vi "Main_Potential-Field_Sim.vi"() -> ()   [LabVIEW 2019]
uses:
  Ctrl/cmd_common.ctl
panel:
  in  "tap":enum32{"Main", "Data"}(tab)
  in  "set goal point":bool
  in  "set start point":bool
  in  "calc potential map":bool
  out "Potential graph":dbl[][](graph)
  in  "Run":bool
  in  "clear":bool
  out "N of obstacles":i32(slide)=8 scale=0.0..20.0
  in  "add obstacle":bool
  in  "Finish":bool
  out "Waypoint":cluster{"rxy":cluster{"x":dbl, "y":dbl}[]}[](graph)=[{"rxy"=[{"x"=9.0, "y"=13.0}]}, {"rxy"=[{"x"=111.0, "y"=90.0}]}, {"rxy"=[{"x"=15.0, "y"=25.0}, {"x"=5.0, "y"=15.0}, {"x"=20.0, "y"=26.0}, {"x"=25.0, "y"=25.0}, {"x"=39.0, "y"=43.0}, {"x"=57.0, "y"=62.0}, {"x"=53.0, "y"=40.0}, {"x"=65.0, "y"=65.0}]}, {"rxy"=[{"x"=65.0, "y"=65.0}]}, {"rxy"=[{"x"=9.0, "y"=13.0}, {"x"=9.5, "y"=13.5}, {"x"=10.0, "y"=14.0}, {"x"=10.5, "y"=14.5}, {"x"=11.0, "y"=15.0}, {"x"=11.5, "y"=15.5}, {"x"=12.0, "y"=16.0}, {"x"=12.5, "y"=16.5}, {"x"=13.0, "y"=17.0}, {"x"=13.5, "y"=17.5}, {"x"=14.0, "y"=18.0}, {"x"=14.5, "y"=18.5}, {"x"=15.0, "y"=19.0}, {"x"=15.5, "y"=19.5}, {"x"=16.0, "y"=20.0}, {"x"=16.5, "y"=20.5}, {"x"=17.0, "y"=21.0}, {"x"=17.5, "y"=21.5}, {"x"=18.0, "y"=22.0}, {"x"=18.5, "y"=22.5}, {"x"=19.0, "y"=23.0}, {"x"=19.5, "y"=23.0}, {"x"=20.0, "y"=23.0}, {"x"=20.5, "y"=23.0}, {"x"=21.0, "y"=23.0}, {"x"=21.5, "y"=23.5}, {"x"=22.0, "y"=24.0}, {"x"=22.5, "y"=24.5}, {"x"=22.5, "y"=25.0}, {"x"=22.5, "y"=25.5}, {"x"=22.5, "y"=26.0}, {"x"=23.0, "y"=26.5}, {"x"=23.5, "y"=27.0}, {"x"=24.0, "y"=27.5}, {"x"=24.5, "y"=28.0}, {"x"=25.0, "y"=28.5}, {"x"=25.5, "y"=29.0}, {"x"=26.0, "y"=29.5}, {"x"=26.5, "y"=30.0}, {"x"=27.0, "y"=30.5}, {"x"=27.5, "y"=31.0}, {"x"=28.0, "y"=31.5}, {"x"=28.5, "y"=32.0}, {"x"=29.0, "y"=32.5}, {"x"=29.5, "y"=33.0}, {"x"=30.0, "y"=33.5}, {"x"=30.5, "y"=34.0}, {"x"=31.0, "y"=34.5}, {"x"=31.5, "y"=35.0}, {"x"=32.0, "y"=35.5}, {"x"=32.5, "y"=36.0}, {"x"=33.0, "y"=36.5}, {"x"=33.5, "y"=37.0}, {"x"=34.0, "y"=37.5}, {"x"=34.5, "y"=38.0}, {"x"=35.0, "y"=38.5}, {"x"=35.5, "y"=39.0}, {"x"=36.0, "y"=39.5}, {"x"=36.5, "y"=40.0}, {"x"=37.0, "y"=40.5}, {"x"=37.5, "y"=40.5}, {"x"=38.0, "y"=40.0}, {"x"=38.5, "y"=40.0}, {"x"=39.0, "y"=40.0}, {"x"=39.5, "y"=40.0}, {"x"=40.0, "y"=40.0}, {"x"=40.5, "y"=40.5}, {"x"=41.0, "y"=41.0}, {"x"=41.5, "y"=41.5}, {"x"=42.0, "y"=42.0}, {"x"=42.5, "y"=42.5}, {"x"=43.0, "y"=43.0}, {"x"=43.5, "y"=43.5}, {"x"=44.0, "y"=44.0}, {"x"=44.5, "y"=44.5}, {"x"=45.0, "y"=45.0}, {"x"=45.5, "y"=45.5}, {"x"=46.0, "y"=46.0}, {"x"=46.5, "y"=46.5}, {"x"=47.0, "y"=47.0}, {"x"=47.5, "y"=47.5}, {"x"=48.0, "y"=48.0}, {"x"=48.5, "y"=48.5}, {"x"=49.0, "y"=49.0}, {"x"=49.5, "y"=49.5}, {"x"=50.0, "y"=50.0}, {"x"=50.5, "y"=50.5}, {"x"=51.0, "y"=51.0}, {"x"=51.5, "y"=51.5}, {"x"=52.0, "y"=52.0}, {"x"=52.5, "y"=52.5}, {"x"=53.0, "y"=53.0}, {"x"=53.5, "y"=53.5}, {"x"=54.0, "y"=54.0}, {"x"=54.5, "y"=54.5}, {"x"=55.0, "y"=55.0}, {"x"=55.5, "y"=55.5}, {"x"=56.0, "y"=56.0}, {"x"=56.5, "y"=56.5}, {"x"=57.0, "y"=57.0}, {"x"=57.5, "y"=57.5}, {"x"=58.0, "y"=58.0}, {"x"=58.5, "y"=58.5}, {"x"=59.0, "y"=59.0}, {"x"=59.5, "y"=59.5}, {"x"=60.0, "y"=60.0}, {"x"=60.5, "y"=60.5}, {"x"=61.0, "y"=61.0}, {"x"=61.5, "y"=61.5}, {"x"=62.0, "y"=62.0}, {"x"=62.5, "y"=62.5}, {"x"=63.0, "y"=63.0}, {"x"=63.5, "y"=62.5}, {"x"=64.0, "y"=62.0}, {"x"=64.5, "y"=62.0}, {"x"=65.0, "y"=62.0}, {"x"=65.5, "y"=62.0}, {"x"=66.0, "y"=62.0}, {"x"=66.5, "y"=62.5}, {"x"=67.0, "y"=63.0}, {"x"=67.5, "y"=63.5}, {"x"=68.0, "y"=64.0}, {"x"=68.5, "y"=64.5}, {"x"=69.0, "y"=65.0}, {"x"=69.5, "y"=65.5}, {"x"=70.0, "y"=66.0}, {"x"=70.5, "y"=66.5}, {"x"=71.0, "y"=67.0}, {"x"=71.5, "y"=67.5}, {"x"=72.0, "y"=68.0}, {"x"=72.5, "y"=68.5}, {"x"=73.0, "y"=69.0}, {"x"=73.5, "y"=69.5}, {"x"=74.0, "y"=70.0}, {"x"=74.5, "y"=70.5}, {"x"=75.0, "y"=71.0}, {"x"=75.5, "y"=71.5}, {"x"=76.0, "y"=72.0}, {"x"=76.5, "y"=72.5}, {"x"=77.0, "y"=73.0}, {"x"=77.5, "y"=73.5}, {"x"=78.0, "y"=74.0}, {"x"=78.5, "y"=74.5}, {"x"=79.0, "y"=75.0}, {"x"=79.5, "y"=75.5}, {"x"=80.0, "y"=76.0}, {"x"=80.5, "y"=76.5}, {"x"=81.0, "y"=77.0}, {"x"=81.5, "y"=77.5}, {"x"=82.0, "y"=78.0}, {"x"=82.5, "y"=78.5}, {"x"=83.0, "y"=79.0}, {"x"=83.5, "y"=79.5}, {"x"=84.0, "y"=80.0}, {"x"=84.5, "y"=80.5}, {"x"=85.0, "y"=81.0}, {"x"=85.5, "y"=81.5}, {"x"=86.0, "y"=82.0}, {"x"=86.5, "y"=82.5}, {"x"=87.0, "y"=83.0}, {"x"=87.5, "y"=83.5}, {"x"=88.0, "y"=84.0}, {"x"=88.5, "y"=84.5}, {"x"=89.0, "y"=85.0}, {"x"=89.5, "y"=85.5}, {"x"=90.0, "y"=86.0}, {"x"=90.5, "y"=86.5}, {"x"=91.0, "y"=87.0}, {"x"=91.5, "y"=87.5}, {"x"=92.0, "y"=88.0}, {"x"=92.5, "y"=88.5}, {"x"=93.0, "y"=89.0}, {"x"=93.5, "y"=89.5}, {"x"=94.0, "y"=90.0}, {"x"=94.5, "y"=90.0}, {"x"=95.0, "y"=90.0}, {"x"=95.5, "y"=90.0}, {"x"=96.0, "y"=90.0}, {"x"=96.5, "y"=90.0}, {"x"=97.0, "y"=90.0}, {"x"=97.5, "y"=90.0}, {"x"=98.0, "y"=90.0}, {"x"=98.5, "y"=90.0}, {"x"=99.0, "y"=90.0}, {"x"=99.5, "y"=90.0}, {"x"=100.0, "y"=90.0}, {"x"=100.5, "y"=90.0}, {"x"=101.0, "y"=90.0}, {"x"=101.5, "y"=90.0}, {"x"=102.0, "y"=90.0}, {"x"=102.5, "y"=90.0}, {"x"=103.0, "y"=90.0}, {"x"=103.5, "y"=90.0}, {"x"=104.0, "y"=90.0}, {"x"=104.5, "y"=90.0}, {"x"=105.0, "y"=90.0}, {"x"=105.5, "y"=90.0}, {"x"=106.0, "y"=90.0}, {"x"=106.5, "y"=90.0}, {"x"=107.0, "y"=90.0}, {"x"=107.5, "y"=90.0}, {"x"=108.0, "y"=90.0}, {"x"=108.5, "y"=90.0}, {"x"=109.0, "y"=90.0}, {"x"=109.5, "y"=90.0}, {"x"=110.0, "y"=90.0}, {"x"=110.5, "y"=90.0}, {"x"=111.0, "y"=90.0}]}]
  in  "global-val":T1={"KP"=5.0, "ETA"=100.0, "AREA_WIDTH"=30.0, "Osc_Det_Len"=3}
  in  "set-val":T2={"start pt"={"x"=0, "y"=10}, "goal pt"={"x"=90, "y"=90}, "grid size"=0.5, "robot radius"=5.0, "obstacles"=[{"x"=15, "y"=25}, {"x"=5, "y"=15}, {"x"=20, "y"=26}, {"x"=25, "y"=25}]}
  out "add point":cluster{i32, i32}={65, 65}
  # "Made by Ybbaek"
  # "Potential Field Simulation"
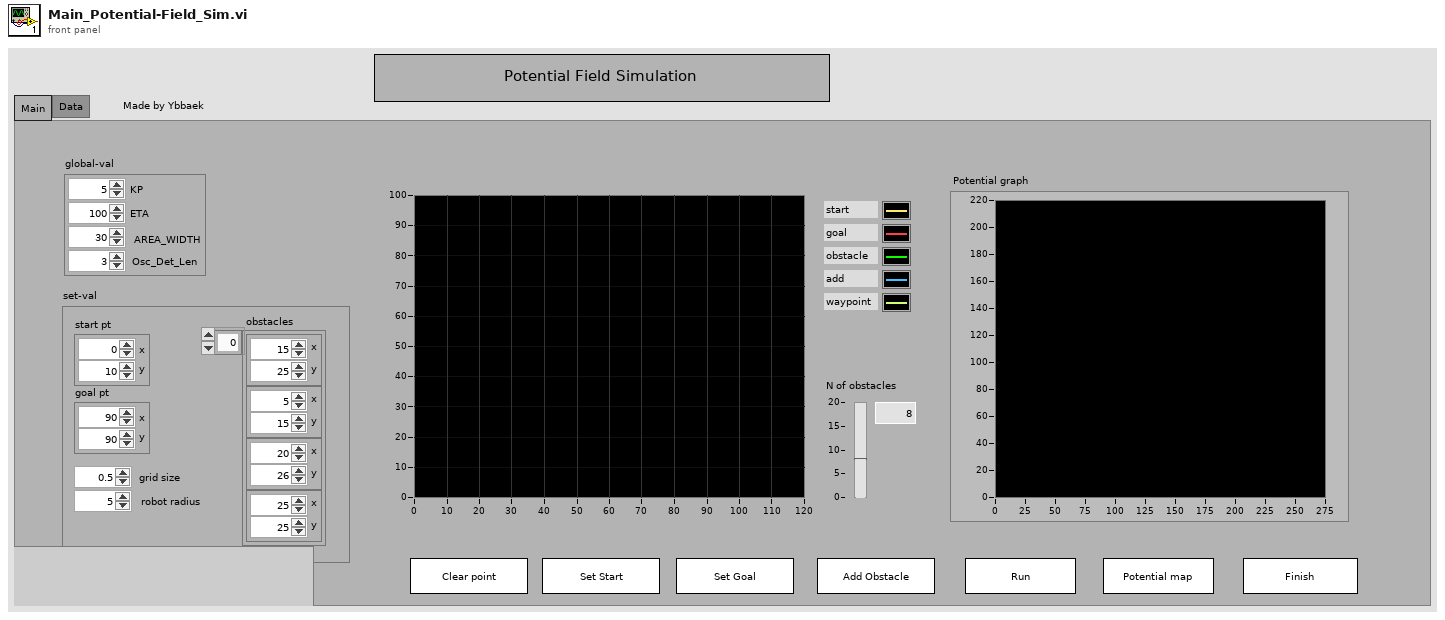
[diagram p1: front panel]
types:
  T1 = cluster{"KP":dbl, "ETA":dbl, "AREA_WIDTH":dbl, "Osc_Det_Len":u32}
  T2 = cluster{"start pt":cluster{"x":i32, "y":i32}, "goal pt":cluster{"x":i32, "y":i32}, "grid size":dbl, "robot radius":dbl, "obstacles":cluster{"x":i32, "y":i32}[]}
  T3 = typedef "cmd_common.ctl" = enum16{"read", "write"}
  T4 = cluster{"start pt":cluster{"x":i32, "y":dbl}, "goal pt":cluster{"x":i32, "y":i32}, "grid size":dbl, "robot radius":dbl, "obstacles":cluster{"x":i32, "y":i32}[]}
  T5 = typedef "NI_Matrix.lvlib/RealMatrix.ctl" = dbl[][]
  T6 = cluster{"delay":dbl, "d":dbl, "rxy":cluster{"x":dbl, "y":dbl}[], "pmap":T5}
  T7 = typedef "LVPoint32TypeDef.ctl" = cluster{"Horizontal":i32, "Vertical":i32}
  T8 = typedef "LVRectTypeDef.ctl" = cluster{"Left":i16, "Top":i16, "Right":i16, "Bottom":i16}
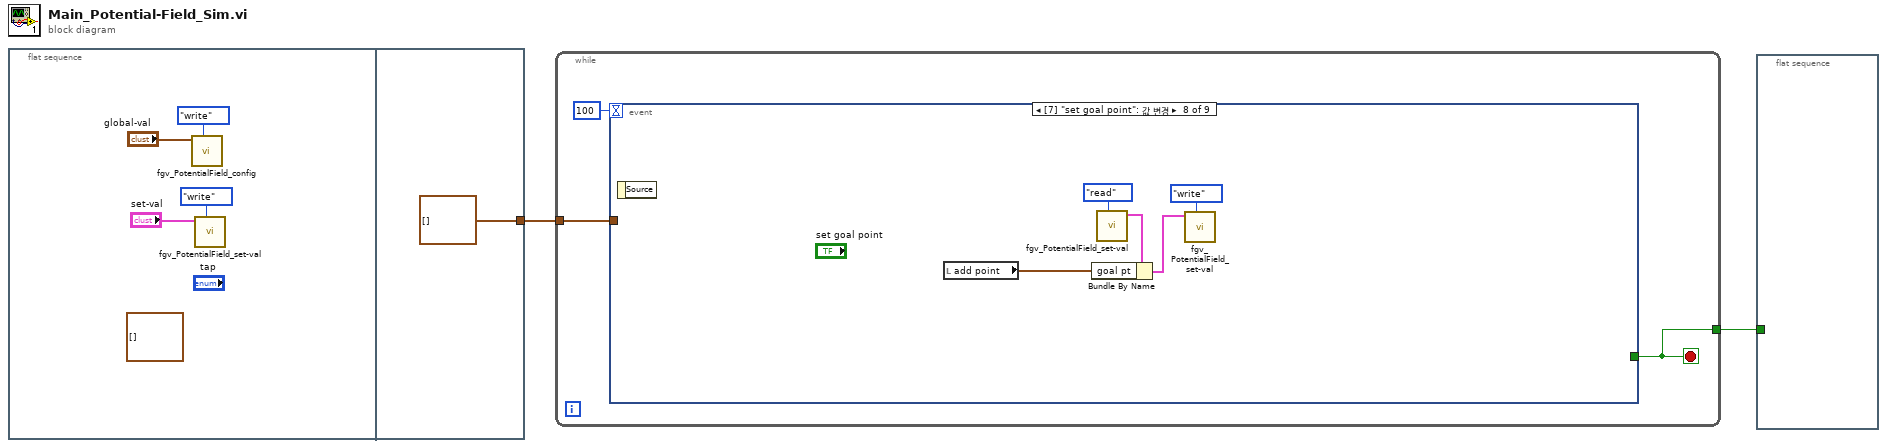
[diagram p0: block diagram]
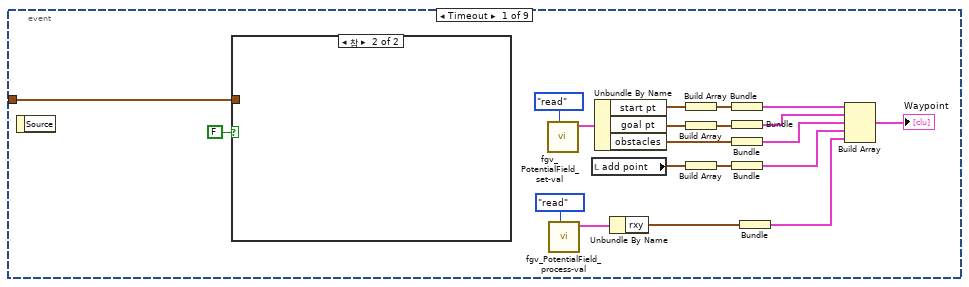
[diagram p2: hidden frame]
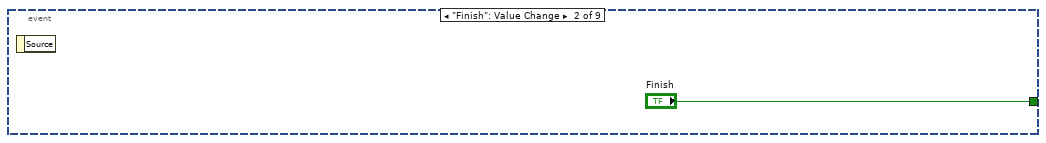
[diagram p4: hidden frame]
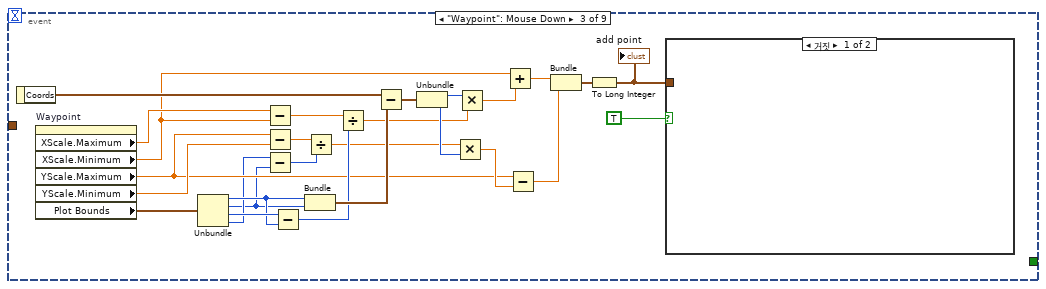
[diagram p5: hidden frame]
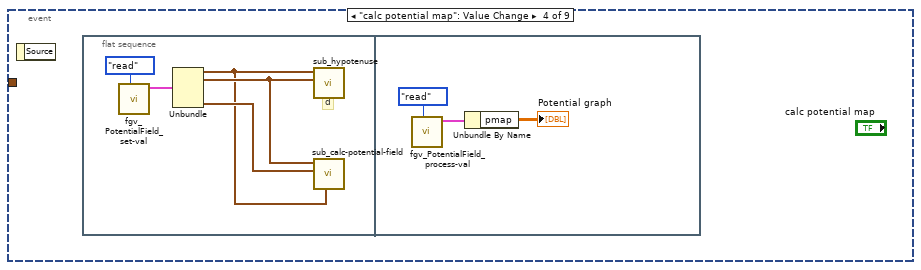
[diagram p7: hidden frame]
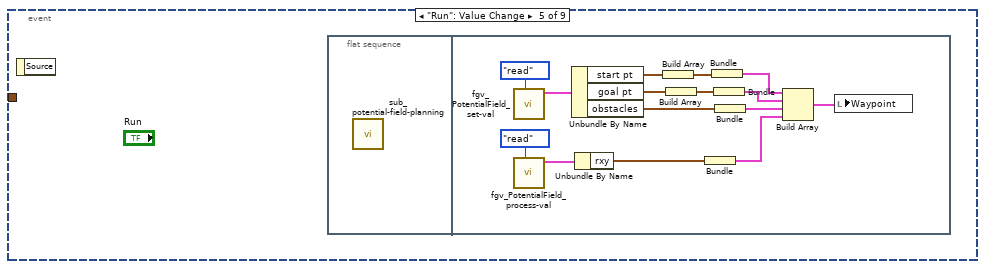
[diagram p8: hidden frame]
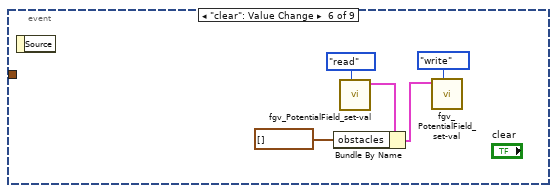
[diagram p9: hidden frame]
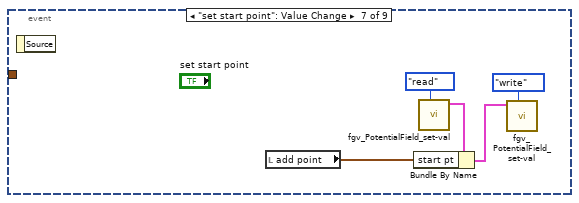
[diagram p10: hidden frame]
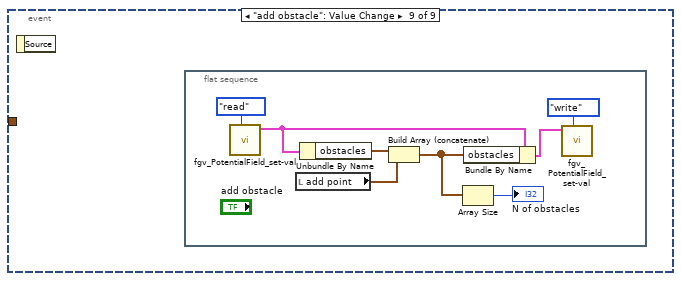
[diagram p11: hidden frame]
diagram:
  n1 = flat-sequence {
    tunnel: [cluster{"X":i32, "Y":i32}[] []] -> w1
    frame #0 {
      (unwired) cluster{i32, i32}[] [] ("add arr")
      n2 = call "fgv_PotentialField_config.vi"("cmd"=cmd_common."write", "pf-val"="global-val") -> ()  [unwired: 9 in, 1 out]
      n3 = call "fgv_PotentialField_set-val.vi"("cmd"=cmd_common."write", "set-val"="set-val") -> ()  [unwired: 9 in, 1 out]
    }
    frame #1 {
    }
  }
  n4 = while {
    tunnel: [w10] -> w2
    tunnel: w1 -> [w9]
    stop <- w10 stop-if-true
    n5 = event shown="[7] \"set goal point\": 값 변경" {
      selector: _ -> [_ _ _ _ _ _ _ _ _]
      dyn-events: _ -> [_ _ _ _ _ _ _ _ _]
      timeout: 100 -> [_ _ _ _ _ _ _ _ _]
      tunnel: [_ "Finish" _ _ _ _ _ _ _] -> w10
      tunnel: w9 -> [w30 _ _ _ _ _ _ _ _]
      event Timeout {
        n6 = event-data() -> ()  [unwired: 1 in, 1 out]
        n7 = case shown="참" FALSE {
          tunnel: w30 -> [_ _]
          frame False {
          }
          frame True {
          }
        }
        n8 = call "fgv_PotentialField_set-val.vi"("cmd"=cmd_common."read") -> ("set-val out"=w26:T4)  [unwired: 10 in]
        n9 = call "fgv_PotentialField_process-val.vi"("cmd"=cmd_common."read") -> ("prcess val out"=w14:T6)  [unwired: 10 in]
        n10 = local read "add point"() -> (w17:cluster{i32, i32})
        n11 = Unbundle By Name(w26) -> ("start pt"=w25:cluster{"x":i32, "y":dbl}, "goal pt"=w22:cluster{"x":i32, "y":i32}, "obstacles"=w18:cluster{"x":i32, "y":i32}[])
        n12 = Unbundle By Name(w14) -> ("rxy"=w13:cluster{"x":dbl, "y":dbl}[])
        n13 = Build Array(w25) -> (w24:cluster{"x":i32, "y":dbl}[])
        n14 = Build Array(w22) -> (w23:cluster{"x":i32, "y":i32}[])
        n15 = Build Array(w17) -> (w16:cluster{i32, i32}[])
        n16 = Bundle(w24) -> (w28:cluster{cluster{"x":i32, "y":dbl}[]})  [unwired: 1 in]
        n17 = Bundle(w23) -> (w21:cluster{cluster{"x":i32, "y":i32}[]})  [unwired: 1 in]
        n18 = Bundle("obstacles"=w18) -> (w19:cluster{"obstacles":cluster{"x":i32, "y":i32}[]})  [unwired: 1 in]
        n19 = Bundle(w16) -> (w15:cluster{cluster{i32, i32}[]})  [unwired: 1 in]
        n20 = Bundle("rxy"=w13) -> (w11:cluster{"rxy":cluster{"x":dbl, "y":dbl}[]})  [unwired: 1 in]
        n21 = Build Array(w28, w21, w19, w15, w11) -> (→"Waypoint":cluster{"rxy":cluster{"x":dbl, "y":dbl}[]}[])
      }
      event "Finish": Value Change {
        n22 = event-data() -> ()  [unwired: 1 in, 1 out]
      }
      event "Waypoint": Mouse Down {
        n23 = event-data() -> ("Coords"=w57:T7)  [unwired: 1 in]
        n24 = property on="Waypoint" class="XYGraph (엄격한)"() -> ("XScale.Maximum"=w55:dbl, "XScale.Minimum"=w47:dbl, "YScale.Maximum"=w39:dbl, "YScale.Minimum"=w42:dbl, "Plot Bounds"=w58:T8)  [unwired: 2 in, 2 out]
        n25 = Unbundle(w58) -> ("Left"=w51:i16, "Top"=w37:i16, "Right"=w52:i16, "Bottom"=w38:i16)
        n26 = Subtract(x=w55, y=w47) -> (x-y=w50:dbl)
        n27 = Subtract(x=w39, y=w42) -> (x-y=w45:dbl)
        n28 = Subtract(x=w38, y=w37) -> (x-y=w44:i16)
        n29 = Subtract(x=w52, y=w51) -> (x-y=w49:i16)
        n30 = Bundle("Left"=w51, "Top"=w37) -> (w56:cluster{"Left":i16, "Top":i16})  [unwired: 1 in]
        n31 = Divide(x=w45, y=w44) -> (x/y=w43:dbl)
        n32 = Divide(x=w50, y=w49) -> (x/y=w35:dbl)
        n33 = Subtract(x=w57, y=w56) -> (x-y=w54:T7)
        n34 = Unbundle(w54) -> ("Horizontal"=w36:i32, "Vertical"=w53:i32)
        n35 = Multiply(x=w43, y=w53) -> (x*y=w41:dbl)
        n36 = Multiply(x=w36, y=w35) -> (x*y=w48:dbl)
        n37 = Add(x=w47, y=w48) -> (x+y=w46:dbl)
        n38 = Subtract(x=w39, y=w41) -> (x-y=w40:dbl)
        n39 = Bundle(w46, w40) -> (w34:cluster{dbl, dbl})  [unwired: 1 in]
        n40 = To Long Integer(number=w34) -> (32bit integer=w33:cluster{i32, i32})
        "add point" <- w33
        n41 = case shown="거짓" TRUE {
          tunnel: w33 -> [_ _]
          frame False {
          }
          frame True {
          }
        }
      }
      event "calc potential map": Value Change {
        n42 = event-data() -> ()  [unwired: 1 in, 1 out]
        n43 = flat-sequence {
          frame #0 {
            # "d"
            n44 = call "fgv_PotentialField_set-val.vi"("cmd"=cmd_common."read") -> ("set-val out"=w62:T4)  [unwired: 10 in]
            n45 = Unbundle(w62) -> ("start pt"=w59:cluster{"x":i32, "y":dbl}, "goal pt"=w60:cluster{"x":i32, "y":i32}, "obstacles"=w61:cluster{"x":i32, "y":i32}[])  [unwired: 2 out]
            n46 = call "sub_hypotenuse.vi"("x2y2"=w60, "x1y1"=w59) -> ()  [unwired: 9 in, 1 out]
            n47 = call "sub_calc-potential-field.vi"("start pt"=w59, "obstacles"=w61, "goal pt"=w60) -> ()  [unwired: 7 in, 2 out]
          }
          frame #1 {
            n48 = call "fgv_PotentialField_process-val.vi"("cmd"=cmd_common."read") -> ("prcess val out"=w66:T6)  [unwired: 10 in]
            n49 = Unbundle By Name(w66) -> ("pmap"=→"Potential graph":T5)
          }
        }
      }
      event "Run": Value Change {
        n50 = event-data() -> ()  [unwired: 1 in, 1 out]
        n51 = flat-sequence {
          frame #0 {
            n52 = call "sub_potential-field-planning.vi"() -> ()  [unwired: 12 in]
          }
          frame #1 {
            n53 = call "fgv_PotentialField_set-val.vi"("cmd"=cmd_common."read") -> ("set-val out"=w80:T4)  [unwired: 10 in]
            n54 = call "fgv_PotentialField_process-val.vi"("cmd"=cmd_common."read") -> ("prcess val out"=w79:T6)  [unwired: 10 in]
            n55 = Unbundle By Name(w80) -> ("start pt"=w74:cluster{"x":i32, "y":dbl}, "goal pt"=w75:cluster{"x":i32, "y":i32}, "obstacles"=w76:cluster{"x":i32, "y":i32}[])
            n56 = Unbundle By Name(w79) -> ("rxy"=w78:cluster{"x":dbl, "y":dbl}[])
            n57 = Build Array(w74) -> (w72:cluster{"x":i32, "y":dbl}[])
            n58 = Build Array(w75) -> (w73:cluster{"x":i32, "y":i32}[])
            n59 = Bundle("rxy"=w78) -> (w67:cluster{"rxy":cluster{"x":dbl, "y":dbl}[]})  [unwired: 1 in]
            n60 = Bundle(w72) -> (w68:cluster{cluster{"x":i32, "y":dbl}[]})  [unwired: 1 in]
            n61 = Bundle(w73) -> (w70:cluster{cluster{"x":i32, "y":i32}[]})  [unwired: 1 in]
            n62 = Bundle("obstacles"=w76) -> (w71:cluster{"obstacles":cluster{"x":i32, "y":i32}[]})  [unwired: 1 in]
            n63 = Build Array(w68, w70, w71, w67) -> (w69:cluster{"rxy":cluster{"x":dbl, "y":dbl}[]}[])
            n64 = local write "Waypoint"(w69) -> ()
          }
        }
      }
      event "clear": Value Change {
        n65 = event-data() -> ()  [unwired: 1 in, 1 out]
        n66 = call "fgv_PotentialField_set-val.vi"("cmd"=cmd_common."read") -> ("set-val out"=w85:T4)  [unwired: 10 in]
        n67 = Bundle By Name(cluster=w85, "obstacles"=cluster{dbl, dbl}[] [] ("add arr")) -> (w86:T4)
        n68 = call "fgv_PotentialField_set-val.vi"("cmd"=cmd_common."write", "set-val"=w86) -> ()  [unwired: 9 in, 1 out]
      }
      event "set start point": Value Change {
        n69 = event-data() -> ()  [unwired: 1 in, 1 out]
        n70 = local read "add point"() -> (w87:cluster{i32, i32})
        n71 = call "fgv_PotentialField_set-val.vi"("cmd"=cmd_common."read") -> ("set-val out"=w90:T4)  [unwired: 10 in]
        n72 = Bundle By Name(cluster=w90, "start pt"=w87) -> (w91:T4)
        n73 = call "fgv_PotentialField_set-val.vi"("cmd"=cmd_common."write", "set-val"=w91) -> ()  [unwired: 9 in, 1 out]
      }
      event "set goal point": Value Change {
        n74 = event-data() -> ()  [unwired: 1 in, 1 out]
        n75 = local read "add point"() -> (w94:cluster{i32, i32})
        n76 = call "fgv_PotentialField_set-val.vi"("cmd"=cmd_common."read") -> ("set-val out"=w95:T4)  [unwired: 10 in]
        n77 = Bundle By Name(cluster=w95, "goal pt"=w94) -> (w96:T4)
        n78 = call "fgv_PotentialField_set-val.vi"("cmd"=cmd_common."write", "set-val"=w96) -> ()  [unwired: 9 in, 1 out]
      }
      event "add obstacle": Value Change {
        n79 = event-data() -> ()  [unwired: 1 in, 1 out]
        n80 = flat-sequence {
          frame #0 {
            n81 = call "fgv_PotentialField_set-val.vi"("cmd"=cmd_common."read") -> ("set-val out"=w101:T4)  [unwired: 10 in]
            n82 = local read "add point"() -> (w98:cluster{i32, i32})
            n83 = Unbundle By Name(w101) -> ("obstacles"=w97:cluster{"x":i32, "y":i32}[])
            n84 = Build Array (concatenate)(w97, w98) -> (w102:cluster{"x":i32, "y":i32}[])
            n85 = Array Size(array=w102) -> (size(s)=→"N of obstacles":i32)
            n86 = Bundle By Name(cluster=w101, "obstacles"=w102) -> (w103:T4)
            n87 = call "fgv_PotentialField_set-val.vi"("cmd"=cmd_common."write", "set-val"=w103) -> ()  [unwired: 9 in, 1 out]
          }
        }
      }
    }
  }
  n88 = flat-sequence {
    tunnel: w2 -> [_]
    frame #0 {
    }
  }
